vi "IFilterClose.vi"(1 "PRIORLib.IFilter":refnum<k7>) -> (0 "error out":errorcluster)   [LabVIEW 2011]
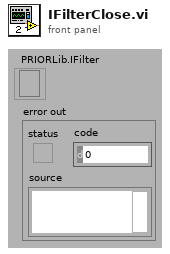
[diagram p1: front panel]
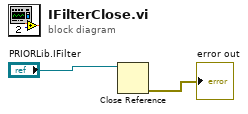
[diagram p0: block diagram]
diagram:
  n1 = Close Reference(reference="PRIORLib.IFilter") -> (error out=→"error out":errorcluster)  [unwired: 1 in]
